vi "New Client Connection.vi"(7 "Client SSL Options (for wss://)":T1={"Check Revocation"=FALSE, "SSL Protocols"=[240]} {"SSL Protocols" items=["None"=0, "Ssl2"=12, "Ssl3"=48, "Tls"=192, "Default"=240, "Tls11"=768, "Tls12"=3072]}, 8 "error in (no error)":errorcluster, 9 "Timeout (5000ms)":i32=5000, 11 "WebSocket URL":string="wss://localhost:7123") -> (0 "error out":errorcluster, 3 "dotNET WS Client out":refnum<class "dotNET WebSocket Client.lvclass">)   [LabVIEW 2013, in "dotNET WebSocket.lvlib" / "dotNET WebSocket Client.lvclass"]
doc: "Opens a new client connection to the given websockets URL using a dotNET SSL socket."
uses:
  dotNET WebSocket Client.lvclass
  dotNET SSL Client/SSL Client Options.ctl
  dotNET SSL Socket/dotNET SSL Socket.lvclass/dotNET SSL Socket.ctl
  dotNET SSL Client/dotNET SSL Client Socket.lvclass
  <vilib>/MediaMongrels Ltd/WebSockets/WebSockets/WebSocket/WebSocket.lvclass/WebSocket.ctl
  <vilib>/MediaMongrels Ltd/WebSockets/WebSockets/WebSocket Client/WebSocket Client.lvclass/WebSocket Client.ctl
  dotNET SSL Socket/Write Check Revocation.vi
  dotNET SSL Socket/Write SSL Protocols.vi
  <vilib>/MediaMongrels Ltd/WebSockets/WebSockets/WebSocket/Write Socket.vi
  <vilib>/MediaMongrels Ltd/WebSockets/WebSockets/WebSocket Client/Write URL.vi
  dotNET TCP Socket/dotNET TCP Socket.lvclass
  <vilib>/MediaMongrels Ltd/WebSockets/WebSockets/WebSocket/WebSocket.lvclass
  <vilib>/MediaMongrels Ltd/WebSockets/WebSockets/WebSocket Client/WebSocket Client.lvclass
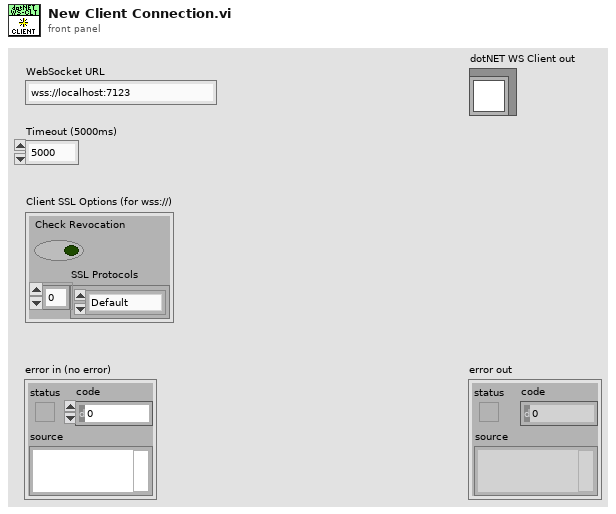
[diagram p1: front panel]
types:
  T1 = typedef "dotNET SSL Socket.lvlib/dotNET SSL Client Socket.lvclass/SSL Client Options.ctl" = cluster{"Check Revocation":bool, "SSL Protocols":i32[]}
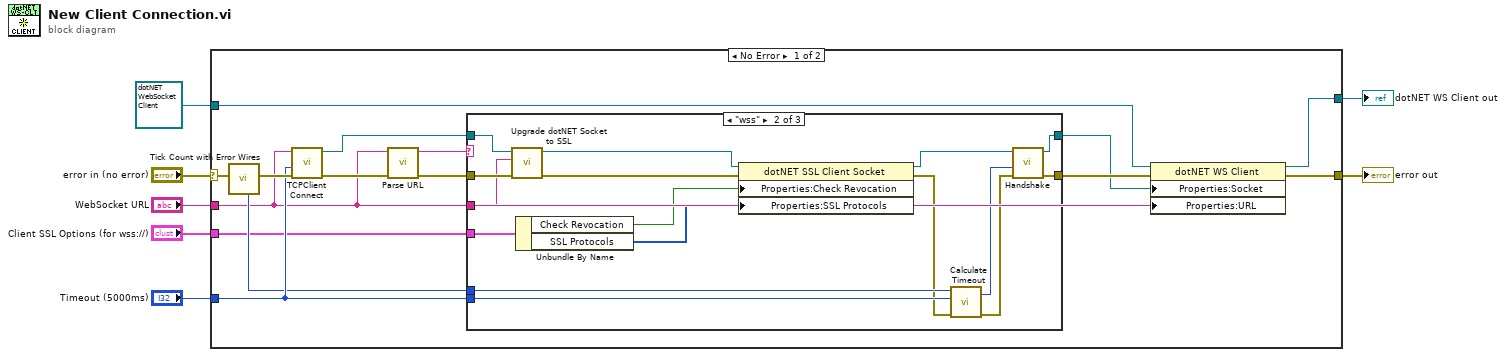
[diagram p0: block diagram]
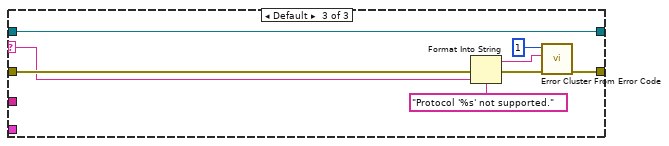
[diagram p3: hidden frame]
diagram:
  n1 = case shown="No Error" "error in (no error)" {
    selector: "error in (no error)" -> [w16 w50]
    tunnel: [w20 w50] -> w6
    tunnel: [w17 w49] -> w3
    tunnel: "WebSocket URL" -> [w10 _]
    tunnel: "Timeout (5000ms)" -> [w14 _]
    tunnel: refnum<class "dotNET WebSocket Client.lvclass"> refnum ("dotNET WS Client out") -> [w19 w49]
    tunnel: "Client SSL Options (for wss://)" -> [w8 _]
    frame No Error {
      n2 = call <vilib>:"Tick Count with Error Wires.vi"("error in (no error)"=w16) -> ("error out"=w15:errorcluster, "millisecond timer value"=w13:u32)  [unwired: 9 in]
      n3 = call "TCPClient Connect.vi"("error in (no error)"=w15, "Timeout (5000ms)"=w14, "Hostname / URL"=w10) -> ("error out"=w12:errorcluster, "dotNET TCP Socket out"=w22:refnum<class "dotNET TCP Socket.lvclass">)  [unwired: 7 in]
      n4 = call <vilib>:"Parse URL.vi"("error in (no error)"=w12, "WebSocket URL"=w10) -> ("error out"=w11:errorcluster, "protocol"=w9:string)  [unwired: 5 in, 3 out]
      n5 = case shown="\"wss\"" w9 {
        selector: w9 -> [_ _ w42]
        tunnel: w22 -> [w24 w40 w48]
        tunnel: w11 -> [w23 w39 w46]
        tunnel: [w23 w38 w47] -> w21
        tunnel: w10 -> [_ w37 _]
        tunnel: [w24 w36 w48] -> w18
        tunnel: w14 -> [_ w35 _]
        tunnel: w13 -> [_ w34 _]
        tunnel: w8 -> [_ w27 _]
        frame "ws" {
        }
        frame "wss" {
          n6 = call "Upgrade dotNET Socket to SSL.vi"("error in (no error)"=w39, "Hostname / URL"=w37, "dotNET TCP Socket in"=w40) -> ("error out"=w33:errorcluster, "dotNET SSL Client Socket out"=w29:refnum<class "dotNET SSL Client Socket.lvclass">)  [unwired: 7 in]
          n7 = Unbundle By Name(w27) -> ("Check Revocation"=w26:bool, "SSL Protocols"=w25:i32[])
          n8 = property class="dotNET SSL Client Socket"(reference=w29, error in=w33, "Properties:Check Revocation"=w26, "Properties:SSL Protocols"=w25) -> (reference out=w28:refnum<class "dotNET SSL Client Socket.lvclass">, error out=w30:errorcluster)
          n9 = call <vilib>:"Calculate Timeout.vi"("error in (no error)"=w30, "timeout ms"=w35, "t0"=w34) -> ("error out"=w32:errorcluster, "new timeout ms"=w31:i32)  [unwired: 6 in, 1 out]
          n10 = call-dynamic "Handshake.vi"("error in (no error)"=w32, "Timeout (5000ms)"=w31, "dotNET SSL Client Socket in"=w28) -> ("error out"=w38:errorcluster, "dotNET SSL Client Socket out"=w36:refnum<class "dotNET SSL Client Socket.lvclass">)  [unwired: 7 in]
        }
        frame Default {
          n11 = Format Into String(format string="Protocol '%s' not supported.", error in=w46, w42) -> (resulting string=w44:string, error out=w45:errorcluster)  [unwired: 1 in]
          n12 = call <vilib>:"Error Cluster From Error Code.vi"("error in (no error)"=w45, "error message (\"\")"=w44, "error code (0)"=1) -> ("error out"=w47:errorcluster)  [unwired: 6 in]
        }
      }
      n13 = property class="dotNET WS Client"(reference=w19, error in=w21, "Properties:Socket"=w18, "Properties:URL"=w10) -> (reference out=w17:refnum<class "dotNET WebSocket Client.lvclass">, error out=w20:errorcluster)
    }
    frame Error {
    }
  }
  "error out" <- w6
  "dotNET WS Client out" <- w3
